vi "NTPModify2.vi"() -> ()   [LabVIEW 2023]
uses:
  <vilib>/Utility/file.llb/Write Delimited Spreadsheet (I64).vi
panel:
  in  "Boolean":bool
  in  "k":i32=8
  in  "const + StdAvr":dbl
  out "My std":dbl[](array[numeric]) format="%#_3g"
  out "Mean":dbl format="%.2f"
  out "Std":dbl format="%#_4g"
  out "Waveform Chart 4":dbl[][](graph) caption="Waveform Chart"
  out "Waveform Chart 3":dbl[][](graph) caption="Waveform Chart"
  out "Waveform Chart 2":u64[][](graph) caption="Waveform Chart"
  out "Waveform Chart":i64[][](graph)
  out "Numeric":i32
  out "last Date":string
  out "AvrStd":dbl[](array[numeric])
  out "tmp64bit":i64[](array[numeric])
  in  "Statistic":bool
  out "StDeviation":dbl[](array[numeric]) format="%#_4g"
  in  "Matches Tab":enum32{"Page 1", "Page 2"}(tab)
  out "Table Control":string[][](table)
  out "appended array":string[](array[string])
  out "Mean by row":dbl[](array[numeric]) format="%.2f"
  out "Variance (xi - x) by row of 6@49":dbl[][](array[numeric])
  out "Last Draw":i64[](array[numeric])
  out "Matches":i32[][](array[numeric])
  out "Matches":i32[](array[numeric])
  out "Last Suppose":i32[][](array[numeric])
  out "Indicator":bool
  in  "Deviation":bool
  in  "Check":bool
  in  "Play":bool
  out "Your Suppose":i32[][](array[numeric])
  in  "Stop":bool
  # "V"
  # "G"
  # "Y"
  # "Last Draw"
  # "Last Suppose"
  # "Last Suppose"
  # "Suppose Graph"
  # "Std Deviation"
  # "6@49"
  # "Your Suppose"
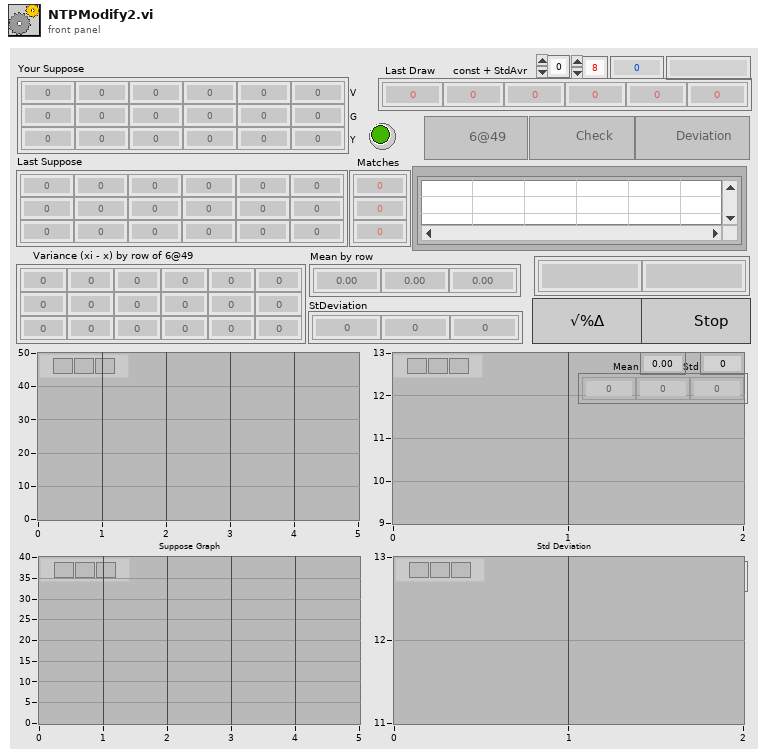
[diagram p1: front panel]
types:
  T1 = enum8{"Enabled", "Disabled", "Disabled and Grayed Out"}
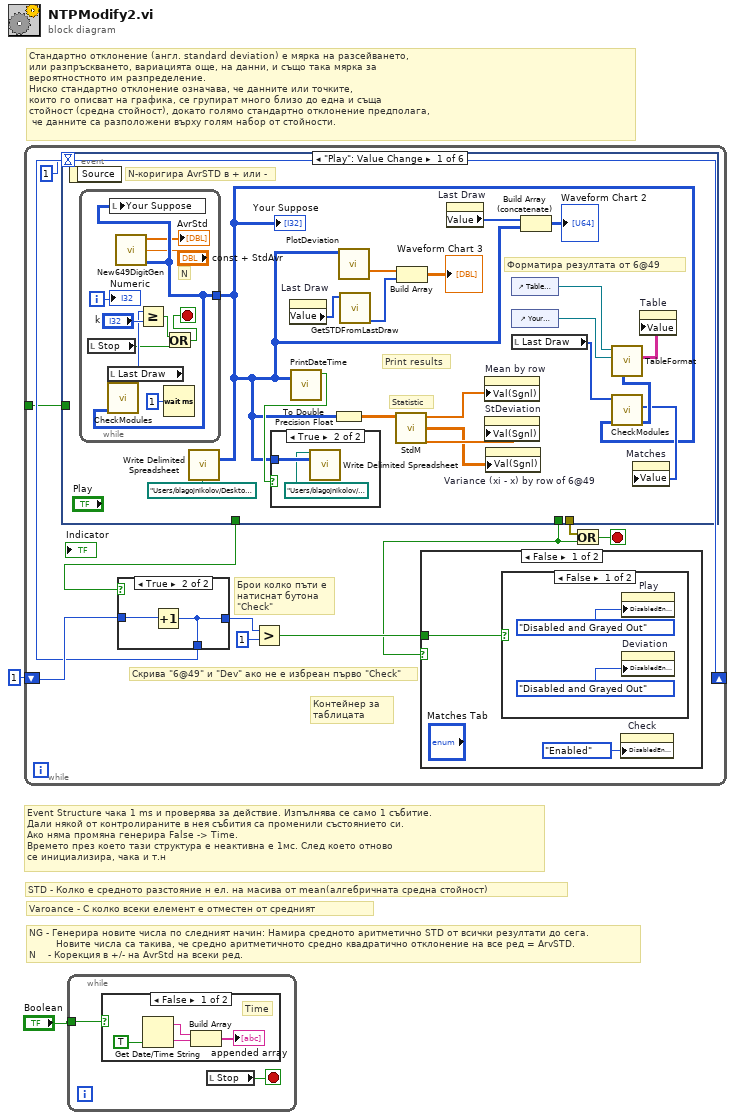
[diagram p0: block diagram]
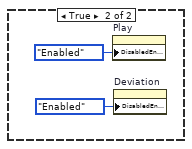
[diagram p4: hidden frame]
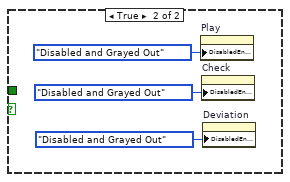
[diagram p5: hidden frame]
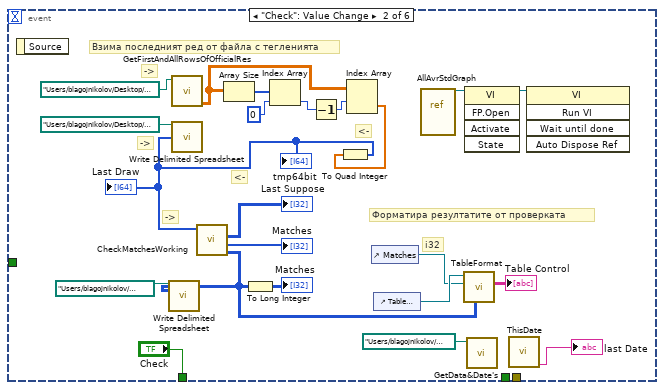
[diagram p7: hidden frame]
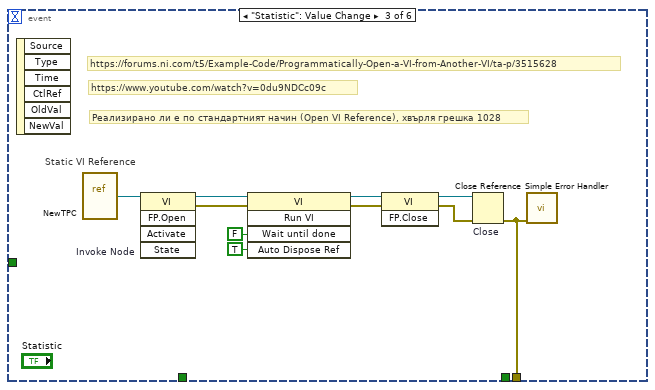
[diagram p8: hidden frame]
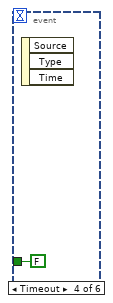
[diagram p9: hidden frame]
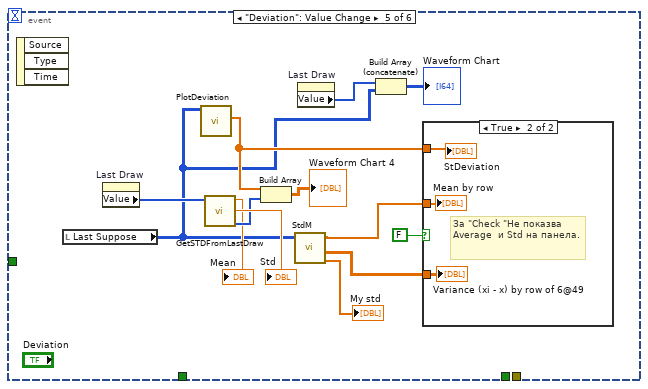
[diagram p10: hidden frame]
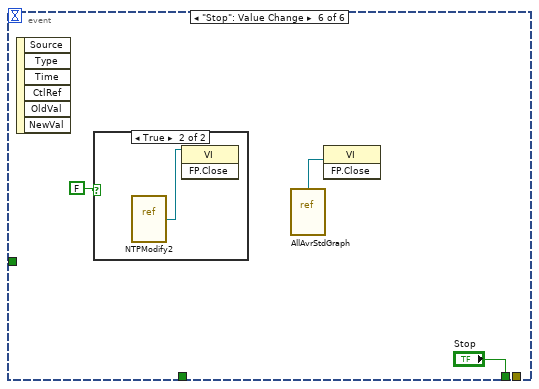
[diagram p12: hidden frame]
diagram:
  # "NG - Генерира новите числа по следният начин: Намира средното аритметично STD от всички резултати до сега.\n         Новите числа са такива, че средно аритметичното средно квадратично отклонение на все ред = ArvSTD. \nN    - Корекция в +/- на AvrStd на всеки ред."
  # "Varoance - С колко всеки елемент е отместен от средният"
  # "STD - Колко е средното разстояние н ел. на масива от mean(алгебричната средна стойност)"
  # "Event Structure чака 1 ms и проверява за действие. Изпълнява се само 1 събитие.\nДали някой от контролираните в нея събития са променили състоянието си.\nАко няма промяна генерира False -> Time.\nВремето през което тази структура е неактивна е 1мс. След което отново\nсе инициализира, чака и т.н"
  # "Стандартно отклонение (англ. standard deviation) е мярка на разсейването, \nили разпръскването, вариацията още, на данни, и също така мярка за \nвероятностното им разпределение. \nНиско стандартно отклонение означава, че данните или точките, \nкоито го описват на графика, се групират много близо до една и съща \nстойност (средна стойност), докато голямо стандартно отклонение предполага,\n че данните са разположени върху голям набор от стойности."
  n1 = while {
    shift-right: [w10] -> _
    shift-left: i64 1 -> [w12]
    tunnel: [w3] -> _
    stop <- w4 stop-if-true
    # "Скрива \"6@49\" и \"Dev\" ако не е избреан първо \"Check\""
    # "Брои колко пъти е\nнатиcнат бутона\n\"Check\""
    # "Контейнер за\nтаблицата"
    n2 = event shown="[0] \"Play\": Value Change" {
      selector: _ -> [_ _ _ _ _ _]
      dyn-events: _ -> [_ _ _ _ _ _]
      timeout: 1 -> [_ _ _ _ _ _]
      tunnel: [_ _ _ FALSE _ _] -> w3
      tunnel: [_ _ _ _ _ "Stop"] -> w6
      tunnel: [_ "Check" _ _ _ _] -> w7
      tunnel: [_ _ w82 _ _ _] -> w5
      event "Play": Value Change {
        # "N-коригира AvrSTD в + или -"
        # "Statistic"
        # "Форматира резултата от 6@49"
        # "Print results"
        n3 = event-data() -> ()  [unwired: 1 in, 1 out]
        n4 = while {
          tunnel: [w54] -> w26
          i -> [w52]
          stop <- w48 stop-if-true
          # "N"
          n5 = local read "Stop"() -> (w50:bool)
          n6 = local read "Last Draw"() -> (w55:i64[])
          n7 = call "New649DigitGen.vi"("const + StdAvr"="const + StdAvr") -> ("2D ResUArr - STD of each row is equal to (Last STD - Avr STD)"=w54:u64[][], "CurrAvrSTDToArr - only six"=→"AvrStd":dbl[])  [unwired: 7 in, 2 out]
          n8 = call "CheckModules.vi"("Your Suppose"=w54, "Last Draw"=w55) -> ("Sum"=w53:i32)  [unwired: 7 in, 2 out]
          n9 = local write "Your Suppose"(w54) -> ()
          n10 = Greater Or Equal?(x=w53, y="k") -> (x >= y?=w51:bool)
          n11 = Wait (ms)(milliseconds to wait=u32 1) -> ()  [unwired: 1 out]
          n12 = Or(x=w51, y=w50) -> (x .or. y?=w48:bool)
          "Numeric" <- w52
        }
        "Your Suppose" <- w26
        n13 = call-poly <vilib>:"Write Delimited Spreadsheet.vi"("file path (dialog if empty)"=path "/Users/blagojnikolov/Desktop/@tmp/tmp649Gen.txt", "2D data"=w26) -> ()  [unwired: 12 in, 2 out]
        n14 = property on="Last Draw" class="Arr (strict)"() -> ("Value"=w37:i64[])  [unwired: 2 in, 2 out]
        n15 = call "PrintDateTime.vi"("2D"=w26) -> ("T button?"=w43:bool)  [unwired: 10 in]
        n16 = case shown="True" w43 {
          tunnel: w26 -> [_ w46]
          frame False {
          }
          frame True {
            n17 = call-poly <vilib>:"Write Delimited Spreadsheet.vi"("file path (dialog if empty)"=path "/Users/blagojnikolov/Desktop/@tmp/archive.txt", "2D data"=w46) -> ()  [unwired: 12 in, 2 out]
          }
        }
        n18 = To Double Precision Float(number=w26) -> (double precision float=w27:dbl[][])
        n19 = call "PlotDeviation.vi"("Array"=w26) -> ("STD"=w40:dbl[])  [unwired: 7 in, 3 out]
        n20 = call "GetSTDFromLastDraw.vi"("Officials Results"=w37) -> ("StdRes array"=w39:u64[])  [unwired: 8 in, 2 out]
        n21 = call "StdM.vi"("2D in"=w27) -> ("1D Std"=w29:dbl[], "[Xi-X]"=w28:dbl[][], "Mean"=w30:dbl[])  [unwired: 6 in, 2 out]
        n22 = Build Array(w40, w39) -> (→"Waveform Chart 3":dbl[][])
        n23 = property on="Last Draw" class="Arr (strict)"() -> ("Value"=w41:i64[])  [unwired: 2 in, 2 out]
        n24 = property on="Mean by row" class="Arr (strict)"("Val(Sgnl)"=w30) -> ()  [unwired: 2 in, 2 out]
        n25 = property on="StDeviation" class="Arr (strict)"("Val(Sgnl)"=w29) -> ()  [unwired: 2 in, 2 out]
        n26 = property on="Variance (xi - x) by row of 6@49" class="Arr (strict)"("Val(Sgnl)"=w28) -> ()  [unwired: 2 in, 2 out]
        n27 = control-ref of="Table Control"() -> (w36:refnum<vi>)
        n28 = control-ref of="Your Suppose"() -> (w32:refnum<vi>)
        n29 = local read "Last Draw"() -> (w31:i64[])
        n30 = Build Array (concatenate)(w41, w26) -> (→"Waveform Chart 2":u64[][])
        n31 = call "CheckModules.vi"("Your Suppose"=w26, "Last Draw"=w31) -> ("Matches"=w34:i32[][], "Matches 2"=w33:i32[])  [unwired: 7 in, 1 out]
        n32 = call "TableFormat.vi"("2D Double Array"=w34, "Arr Refnum"=w32, "Table in"=w36) -> ("TxtArray"=w35:string[][])  [unwired: 8 in]
        n33 = property on="Matches" class="Arr (strict)"("Value"=w33) -> ()  [unwired: 2 in, 2 out]
        n34 = property on="Table" class="Tbl (strict)"("Value"=w35) -> ()  [unwired: 2 in, 2 out]
      }
      event "Check": Value Change {
        # "->"
        # "->"
        # "->"
        # "<-"
        # "<-"
        # "Взима последният ред от файла с тегленията"
        # "Форматира резултатите от проверката"
        # "i32"
        n35 = event-data() -> ()  [unwired: 1 in, 1 out]
        n36 = call "GetFirstAndAllRowsOfOfficialRes.vi"("file (use dialog)"=path "/Users/blagojnikolov/Desktop/@tmp/results.txt" ("file path (dialog if empty)")) -> ("All Officials Result"=w70:dbl[][])  [unwired: 8 in, 2 out]
        n37 = Array Size(array=w70) -> (size(s)=w68:i32[])
        n38 = Index Array(array=w68, index=0) -> (element=w69:i32)
        n39 = Decrement(x=w69) -> (x-1=w67:i32)
        n40 = Index Array "Index Array"(array=w70, index (row)=w67) -> (element=w66:dbl[])  [unwired: 1 in]
        n41 = To Quad Integer(1:w66) -> (0:w65:i64[])
        "Last Draw" <- w65
        "tmp64bit" <- w65
        n42 = call-poly <vilib>:"Write Delimited Spreadsheet.vi"("file path (dialog if empty)"=path "/Users/blagojnikolov/Desktop/@tmp/officialResults.txt", "1D data"=w65) -> ()  [unwired: 12 in, 2 out]
        n43 = call "CheckMatchesWorking.vi"("Последен тираж"=w65) -> (0:w64:i64[][], "Съвпадения"=→"Matches":i32[], "Залози"=→"Last Suppose":i32[][])  [unwired: 7 in, 1 out]
        n44 = call-poly <vilib>:"Write Delimited Spreadsheet.vi"("file path (dialog if empty)"=path "/Users/blagojnikolov/Desktop/@tmp/matches.txt", "2D data"=w64) -> ()  [unwired: 12 in, 2 out]
        n45 = To Long Integer(number=w64) -> (32bit integer=→"Matches":i32[][])
        n46 = control-ref of="Matches"() -> (w74:refnum<vi>)
        n47 = control-ref of="Table Control"() -> (w76:refnum<vi>)
        n48 = vi-ref "AllAvrStdGraph.vi"() -> (w59:refnum<vi>)
        n49 = call "TableFormat.vi"("2D Double Array"=w64, "Arr Refnum"=w74, "Table in"=w76) -> ("TxtArray"=→"Table Control":string[][])  [unwired: 8 in]
        n50 = invoke on="Invoke Node" class="VI" method="FP.Open"(reference=w59) -> (reference out=w58:refnum<vi>)  [unwired: 4 in, 4 out]
        n51 = call "GetData&Date's.vi"("file: (fromSite.txt)"=path "/Users/blagojnikolov/Desktop/@tmp/fromSite.txt" ("file (use dialog)")) -> ()  [unwired: 8 in, 3 out]
        n52 = call "ThisDate.vi"() -> ("this.Date"=→"last Date":string)  [unwired: 11 in]
        n53 = invoke class="VI" method="Run VI"(reference=w58) -> ()  [unwired: 4 in, 5 out]
      }
      event "Statistic": Value Change {
        # "Static VI Reference"
        # "Реализирано ли е по стандартният начин (Open VI Reference), хвърля грешка 1028"
        # "https://www.youtube.com/watch?v=0du9NDCc09c"
        # "https://forums.ni.com/t5/Example-Code/Programmatically-Open-a-VI-from-Another-VI/ta-p/3515628"
        n54 = event-data() -> ()  [unwired: 1 in, 6 out]
        n55 = vi-ref "NewTPC.vi"() -> (w81:refnum<vi>)
        n56 = invoke on="Invoke Node" class="VI" method="FP.Open"(reference=w81) -> (reference out=w89:refnum<vi>, error out=w88:errorcluster)  [unwired: 4 in, 3 out]
        n57 = invoke class="VI" method="Run VI"(reference=w89, error in=w88, "Wait until done"=TRUE ("Wait Until Done"), "Auto Dispose Ref"=FALSE ("Auto Dispose Reference")) -> (reference out=w85:refnum<vi>, error out=w84:errorcluster)  [unwired: 1 in, 3 out]
        n58 = invoke class="VI" method="FP.Close"(reference=w85, error in=w84) -> (reference out=w80:refnum<vi>, error out=w83:errorcluster)  [unwired: 1 in, 1 out]
        n59 = Close Reference "Close"(reference=w80, error in (no error)=w83) -> (error out=w82:errorcluster)
        n60 = call <vilib>:"Simple Error Handler.vi"("error in (no error)"=w82) -> ()  [unwired: 4 in, 5 out]
      }
      event Timeout {
        n61 = event-data() -> ()  [unwired: 1 in, 3 out]
      }
      event "Deviation": Value Change {
        n62 = event-data() -> ()  [unwired: 1 in, 3 out]
        n63 = local read "Last Suppose"() -> (w94:i32[][])
        n64 = property on="Last Draw" class="Arr (strict)"() -> ("Value"=w101:i64[])  [unwired: 2 in, 2 out]
        n65 = call "PlotDeviation.vi"("Array"=w94) -> ("STD"=w97:dbl[])  [unwired: 7 in, 3 out]
        n66 = call "GetSTDFromLastDraw.vi"("Officials Results"=w101) -> ("StdRes array"=w98:u64[], "STD"=→"Std":dbl, "Mean"=→"Mean":dbl)  [unwired: 8 in]
        n67 = Build Array(w97, w98) -> (→"Waveform Chart 4":dbl[][])
        n68 = call "StdM.vi"("2D in"=w94) -> ("1D Std"=→"My std":dbl[], "[Xi-X]"=w92:dbl[][], "Mean"=w93:dbl[])  [unwired: 6 in, 2 out]
        n69 = property on="Last Draw" class="Arr (strict)"() -> ("Value"=w102:i64[])  [unwired: 2 in, 2 out]
        n70 = Build Array (concatenate)(w102, w94) -> (→"Waveform Chart":i64[][])
        n71 = case shown="True" FALSE {
          tunnel: w92 -> [_ w106]
          tunnel: w97 -> [_ w105]
          tunnel: w93 -> [_ w104]
          frame False {
          }
          frame True {
            # "За \"Check \"Не показва Average  и Std на панела."
            "Variance (xi - x) by row of 6@49" <- w106
            "Mean by row" <- w104
            "StDeviation" <- w105
          }
        }
      }
      event "Stop": Value Change {
        n72 = event-data() -> ()  [unwired: 1 in, 6 out]
        n73 = case shown="True" FALSE {
          frame False {
          }
          frame True {
            n74 = vi-ref "NTPModify2.vi"() -> (w110:refnum<vi>)
            n75 = invoke on="Invoke Node" class="VI" method="FP.Close"(reference=w110) -> ()  [unwired: 2 in, 3 out]
          }
        }
        n76 = vi-ref "AllAvrStdGraph.vi"() -> (w108:refnum<vi>)
        n77 = invoke on="Invoke Node" class="VI" method="FP.Close"(reference=w108) -> ()  [unwired: 2 in, 3 out]
      }
    }
    n78 = case shown="True" w7 {
      tunnel: [w14 w15] -> w11
      tunnel: [w14 w15] -> w10
      tunnel: w12 -> [w14 w16]
      frame False {
      }
      frame True {
        n79 = Increment(x=w16) -> (x+1=w15:i64)
      }
    }
    n80 = Greater?(x=w11, y=i64 1) -> (0:w13:bool)
    n81 = case shown="False" w6 {
      tunnel: w13 -> [w17 _]
      frame False {
        n82 = case shown="False" w17 {
          frame False {
            n83 = property on="Play" class="Bool"("DisabledEnum"=T1."Disabled and Grayed Out" ("Disabled")) -> ()  [unwired: 2 in, 2 out]
            n84 = property on="Deviation" class="Bool"("DisabledEnum"=T1."Disabled and Grayed Out" ("Disabled")) -> ()  [unwired: 2 in, 2 out]
          }
          frame True {
            n85 = property on="Play" class="Bool"("DisabledEnum"=T1."Enabled" ("Disabled")) -> ()  [unwired: 2 in, 2 out]
            n86 = property on="Deviation" class="Bool"("DisabledEnum"=T1."Enabled" ("Disabled")) -> ()  [unwired: 2 in, 2 out]
          }
        }
        n87 = property on="Check" class="Bool"("DisabledEnum"=T1."Enabled" ("Disabled")) -> ()  [unwired: 2 in, 2 out]
      }
      frame True {
        n88 = property on="Play" class="Bool"("DisabledEnum"=T1."Disabled and Grayed Out" ("Disabled")) -> ()  [unwired: 2 in, 2 out]
        n89 = property on="Check" class="Bool"("DisabledEnum"=T1."Disabled and Grayed Out" ("Disabled")) -> ()  [unwired: 2 in, 2 out]
        n90 = property on="Deviation" class="Bool"("DisabledEnum"=T1."Disabled and Grayed Out" ("Disabled")) -> ()  [unwired: 2 in, 2 out]
      }
    }
    n91 = Or(x=w5, y=w6) -> (x .or. y?=w4:bool)
  }
  n92 = while {
    tunnel: "Boolean" -> [w112]
    stop <- w111 stop-if-true
    n93 = case shown="False" w112 {
      frame False {
        # "Time"
        n94 = Get Date/Time String(want seconds? (F)=TRUE) -> (date string=w114:string, time string=w115:string)  [unwired: 2 in]
        n95 = Build Array(w114, w115) -> (→"appended array":string[])
      }
      frame True {
      }
    }
    n96 = local read "Stop"() -> (w111:bool)
  }
